vi "TAT-Main.vi"() -> ()   [LabVIEW 2017]
panel:
  in  "Modify SN":bool
  in  "PRINT":bool
  in  "Torque IO Status":bool
  in  "Ass IO Status":bool
  in  "Recipe":bool
  out "error out":errorcluster
  in  "Logout":bool
  in  "Stop":bool
  in  "Create Login":bool
  in  "Reports":bool
  in  "Start":bool
  out "Time":string
  out "Date":string
  in  "Login":bool
  # "RBC ORVM- TRACEABILITY, SCANNING & BARCODE PRINTING"
  # "KAPSE SONS ROBOTICS\n& AUTOMATION"
  # "Contact:-- +91 9325640282"
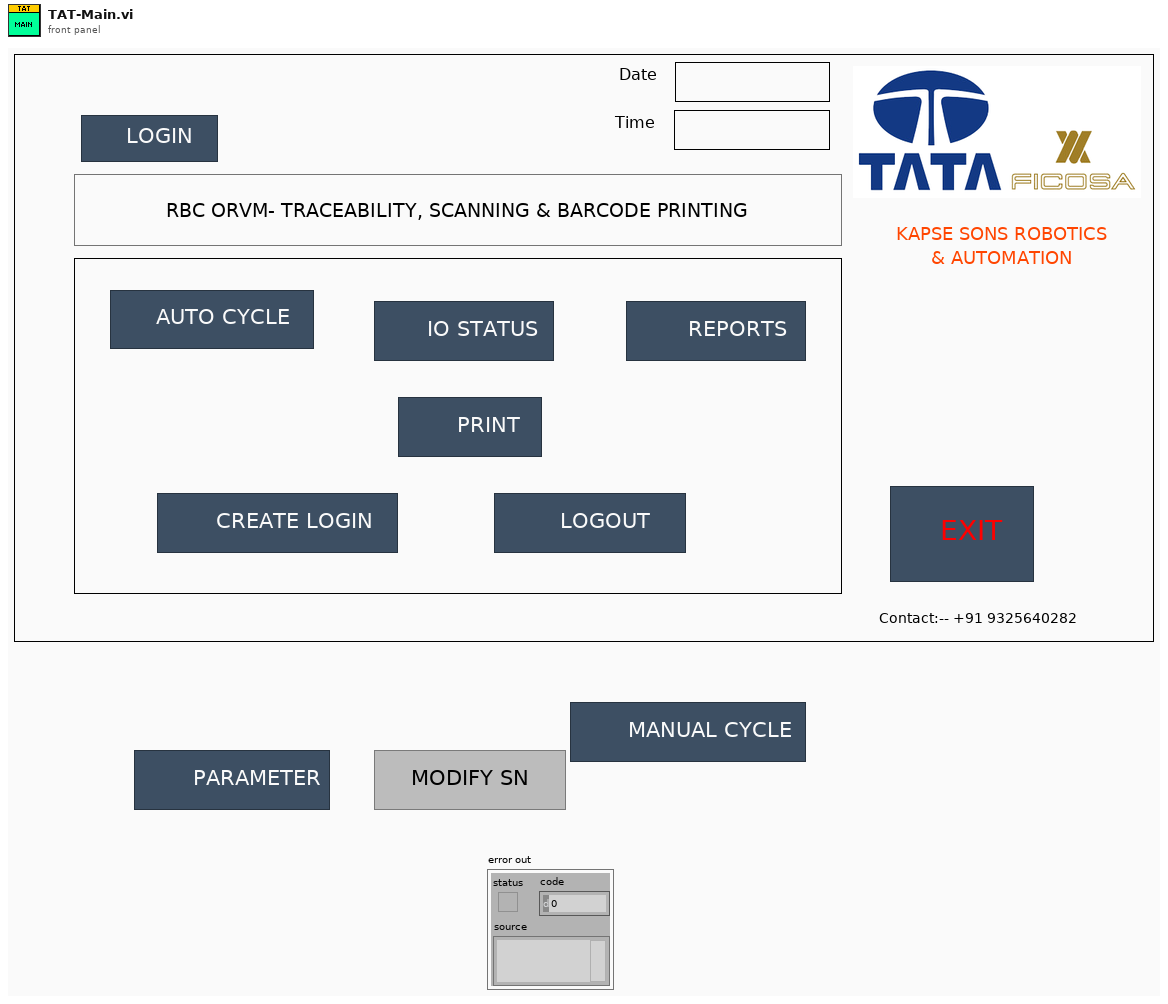
[diagram p1: front panel]
types:
  T1 = enum8{"Enabled", "Disabled", "Disabled and Grayed Out"}
  T2 = enum32{"Invalid", "Standard", "Closed", "Hidden", "Minimized", "Maximized"}
  T3 = enum32{"invalid app kind", "Development System", "Run Time System", "Student Edition", "Embedded LabVIEW", "Evaluation", "Custom"}
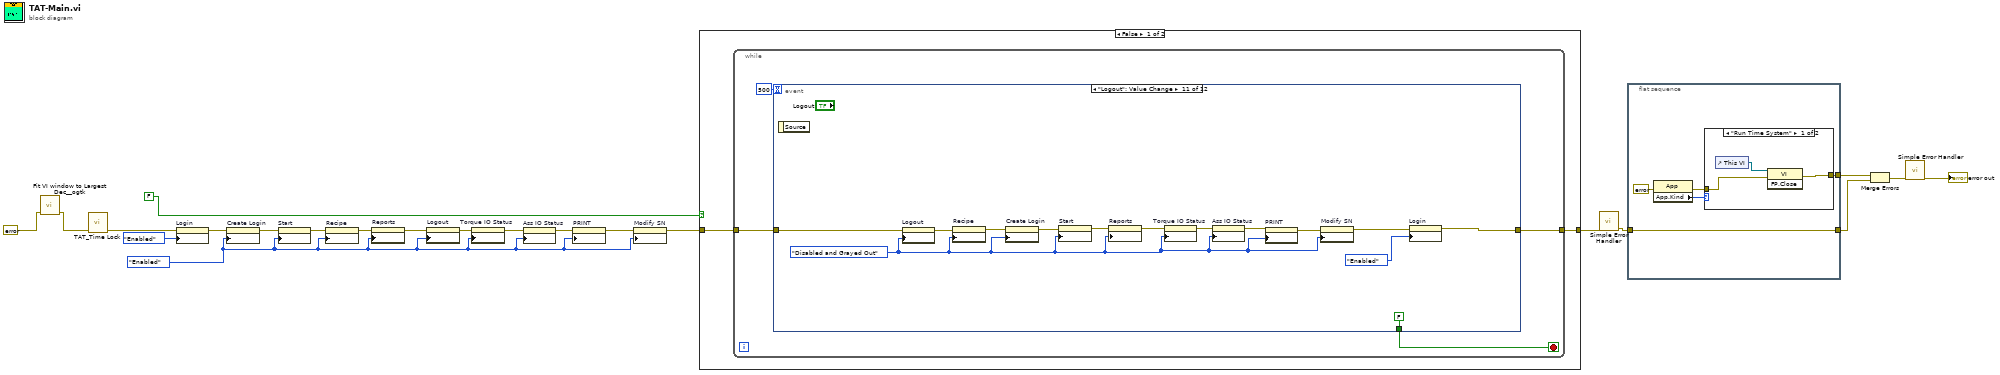
[diagram p0: block diagram]
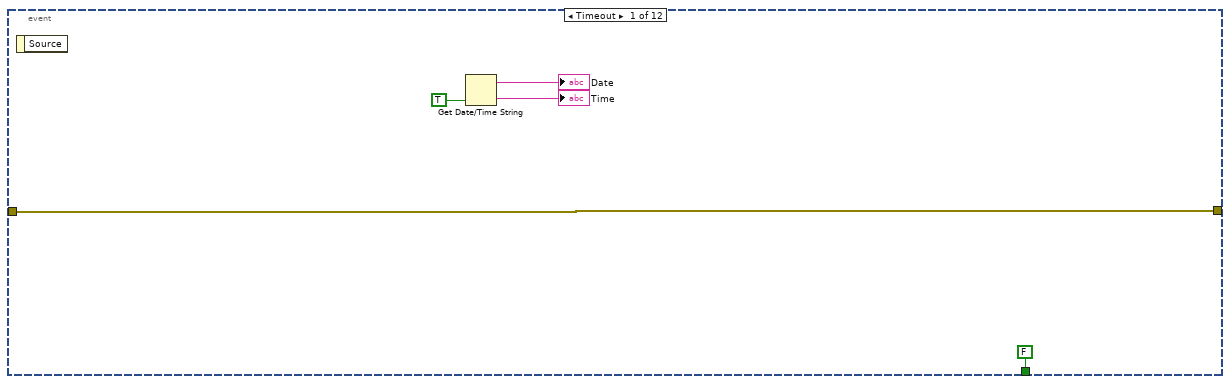
[diagram p3: hidden frame]
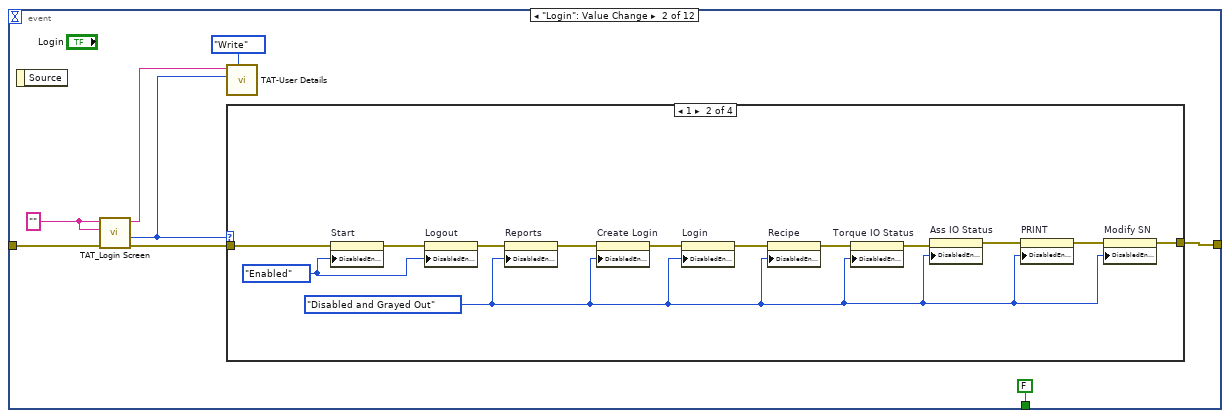
[diagram p4: hidden frame]
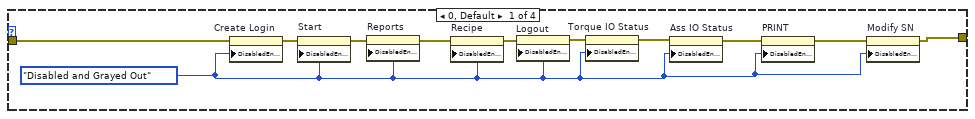
[diagram p5: hidden frame]
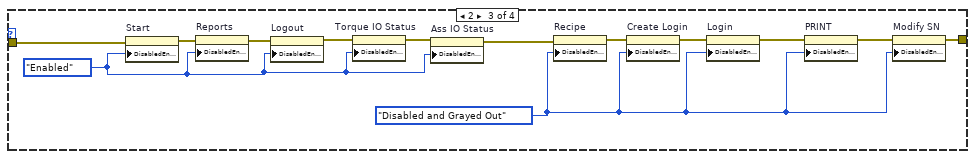
[diagram p6: hidden frame]
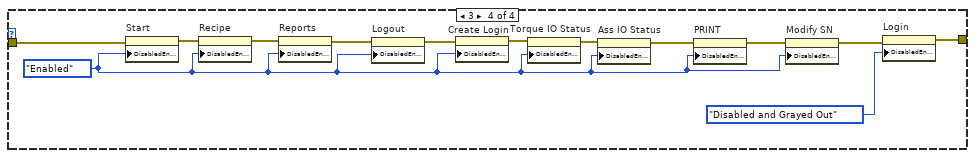
[diagram p7: hidden frame]
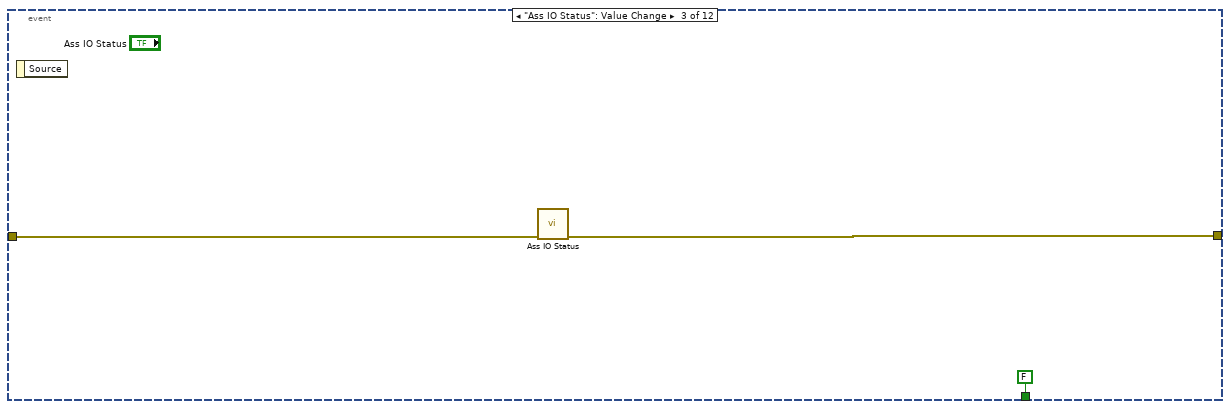
[diagram p8: hidden frame]
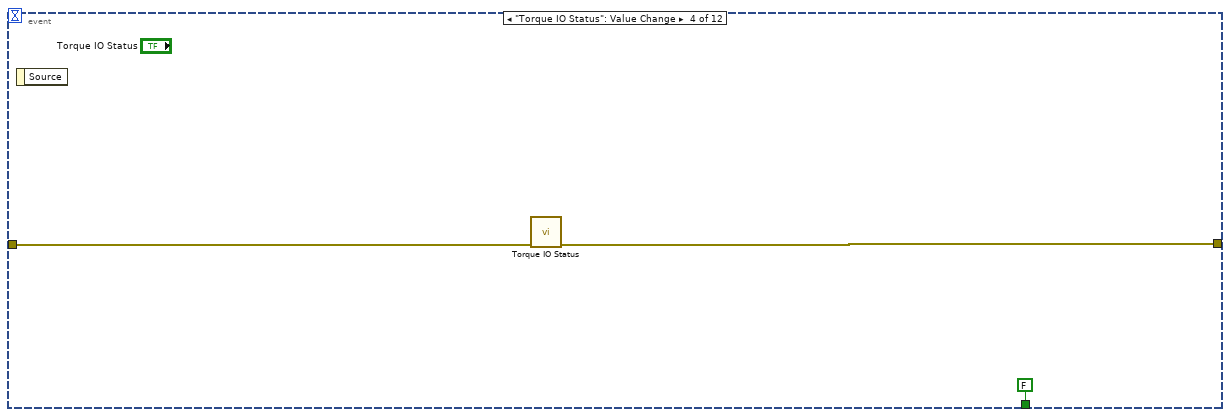
[diagram p9: hidden frame]
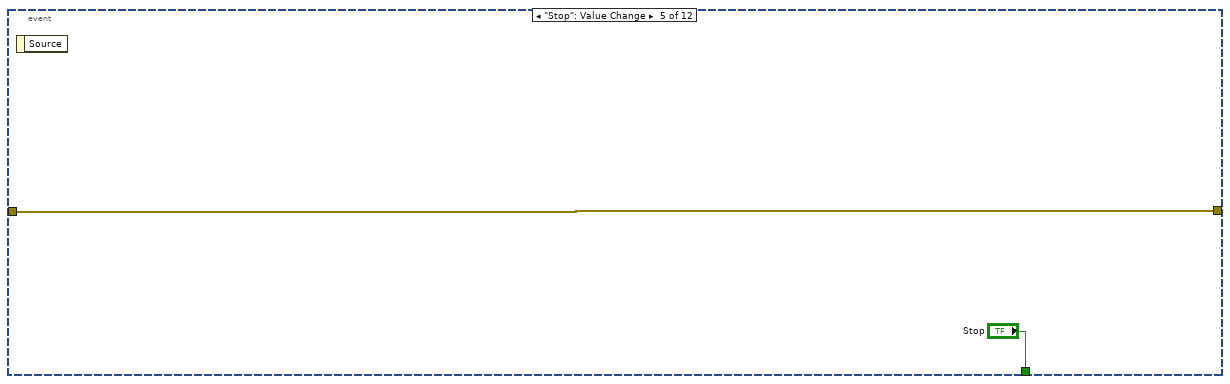
[diagram p10: hidden frame]
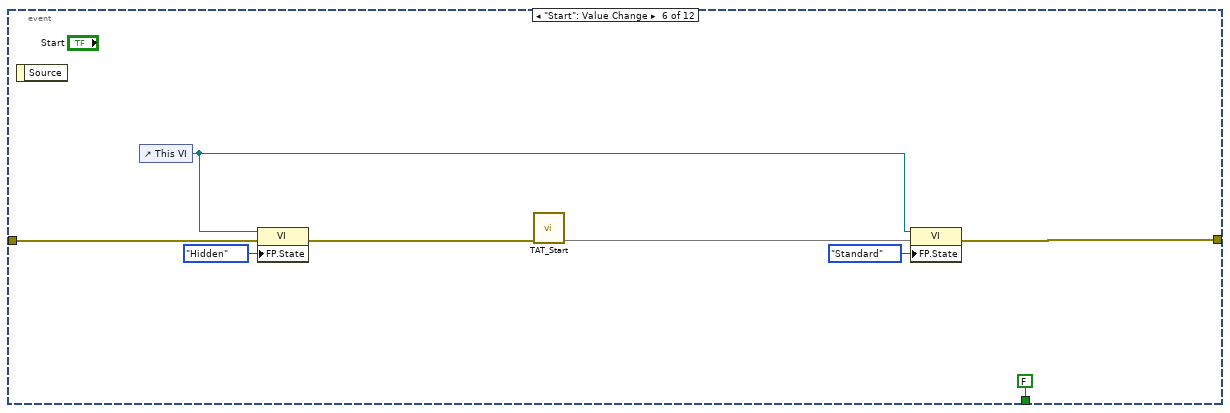
[diagram p11: hidden frame]
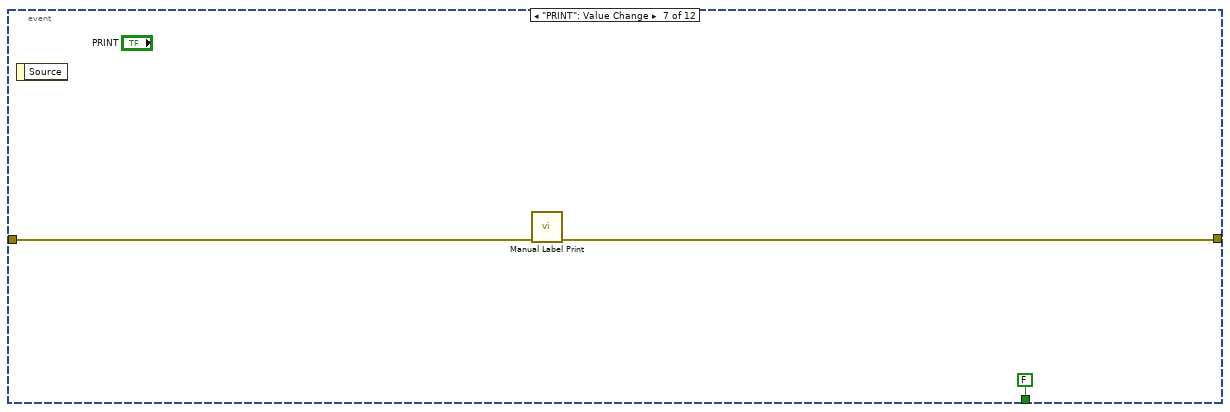
[diagram p12: hidden frame]
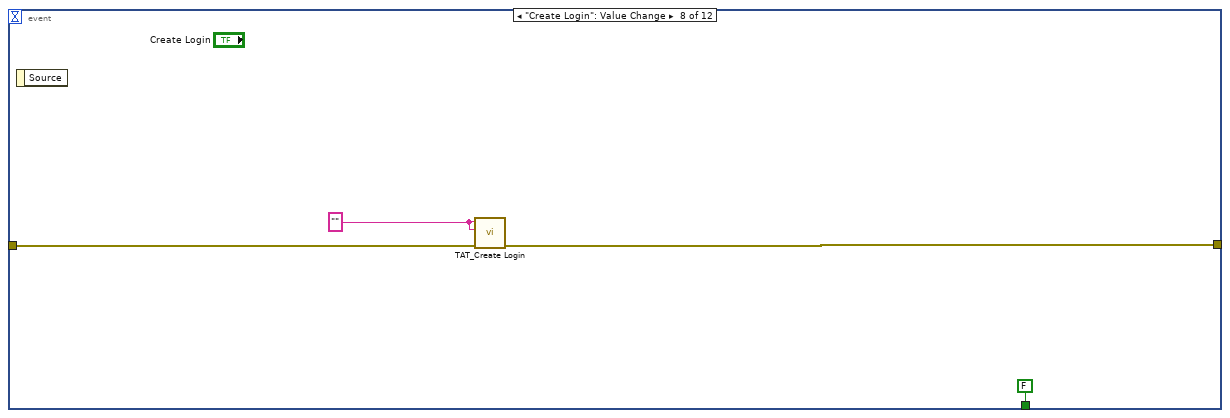
[diagram p13: hidden frame]
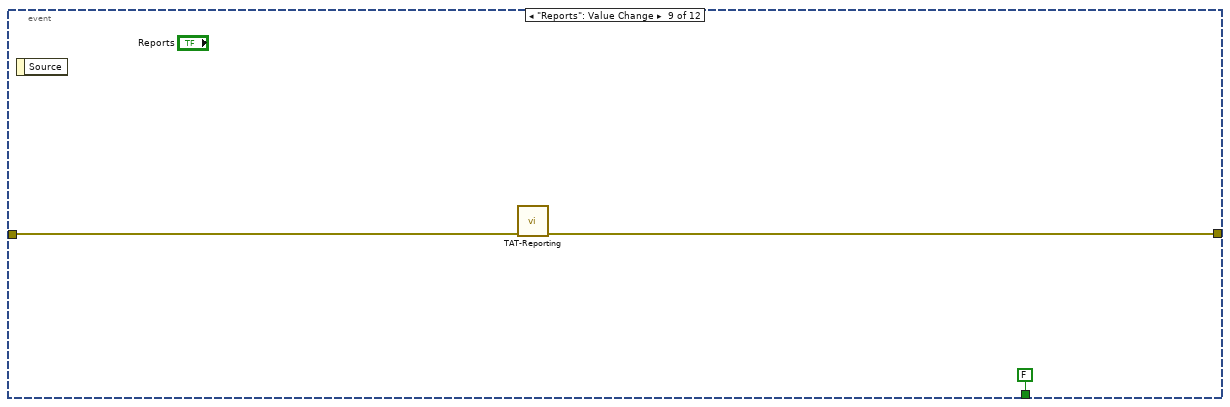
[diagram p14: hidden frame]
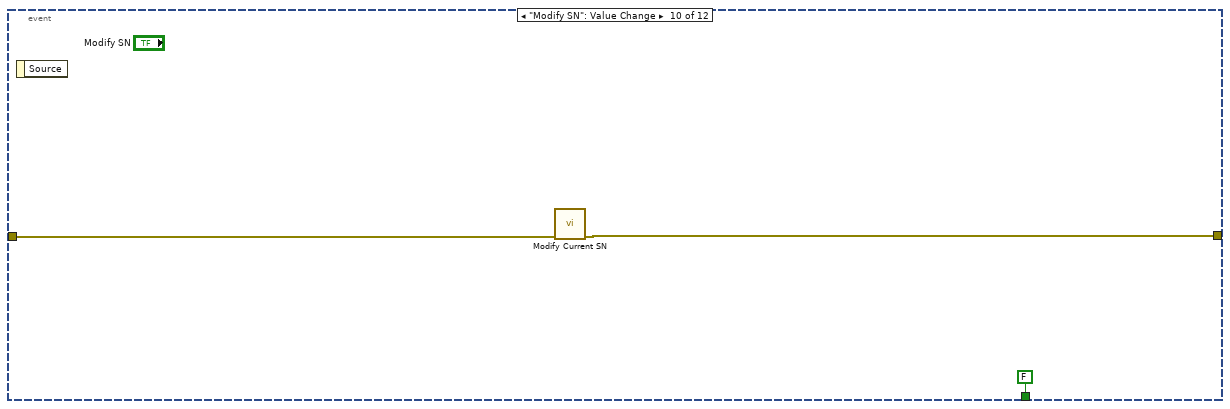
[diagram p15: hidden frame]
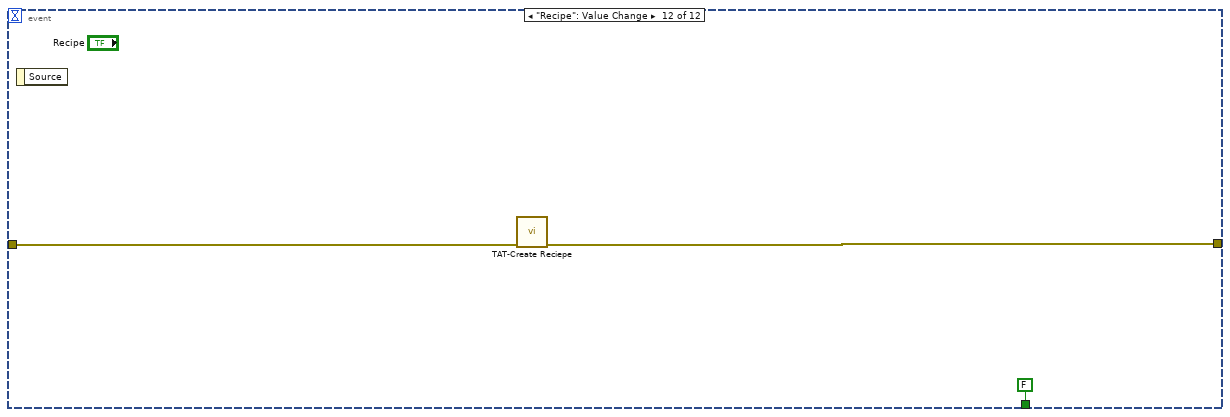
[diagram p16: hidden frame]
diagram:
  w4 = T1."Enabled" ("Disabled")
  n1 = call <userlib>:"Fit VI window to Largest Dec__ogtk.vi"("error in (no error)"=errorcluster {"status"=FALSE, "code"=0, "source"=""} ("error constant")) -> ("error out"=w1:errorcluster)  [unwired: 5 in, 1 out]
  n2 = call "TAT_Time Lock.vi"("error in"=w1) -> ("error out"=w16:errorcluster)  [unwired: 9 in, 1 out]
  n3 = property on="Login" class="Bool"(error in=w16, "DisabledEnum"=T1."Enabled" ("Disabled")) -> (error out=w15:errorcluster)  [unwired: 1 in, 1 out]
  n4 = property on="Create Login" class="Bool"(error in=w15, "DisabledEnum"=w4) -> (error out=w21:errorcluster)  [unwired: 1 in, 1 out]
  n5 = property on="Start" class="Bool"(error in=w21, "DisabledEnum"=w4) -> (error out=w11:errorcluster)  [unwired: 1 in, 1 out]
  n6 = property on="Recipe" class="Bool"(error in=w11, "DisabledEnum"=w4) -> (error out=w10:errorcluster)  [unwired: 1 in, 1 out]
  n7 = property on="Reports" class="Bool"(error in=w10, "DisabledEnum"=w4) -> (error out=w13:errorcluster)  [unwired: 1 in, 1 out]
  n8 = property on="Logout" class="Bool"(error in=w13, "DisabledEnum"=w4) -> (error out=w9:errorcluster)  [unwired: 1 in, 1 out]
  n9 = property on="Torque IO Status" class="Bool"(error in=w9, "DisabledEnum"=w4) -> (error out=w8:errorcluster)  [unwired: 1 in, 1 out]
  n10 = property on="Ass IO Status" class="Bool"(error in=w8, "DisabledEnum"=w4) -> (error out=w7:errorcluster)  [unwired: 1 in, 1 out]
  n11 = property on="PRINT" class="Bool"(error in=w7, "DisabledEnum"=w4) -> (error out=w6:errorcluster)  [unwired: 1 in, 1 out]
  n12 = property on="Modify SN" class="Bool"(error in=w6, "DisabledEnum"=w4) -> (error out=w5:errorcluster)  [unwired: 1 in, 1 out]
  n13 = case shown="False" FALSE {
    tunnel: w5 -> [w24 w138]
    tunnel: [w23 w138] -> w22
    frame False {
      n14 = while {
        tunnel: w24 -> [w27]
        tunnel: [w26] -> w23
        stop <- w25 stop-if-true
        n15 = event shown="[10] \"Logout\": Value Change" {
          selector: _ -> [_ _ _ _ _ _ _ _ _ _ _ _]
          dyn-events: _ -> [_ _ _ _ _ _ _ _ _ _ _ _]
          timeout: 500 -> [_ _ _ _ _ _ _ _ _ _ _ _]
          tunnel: w27 -> [w31 w41 w94 w96 w98 w105 w109 w114 w117 w120 w131 w137]
          tunnel: [w31 w39 w93 w95 w98 w102 w108 w113 w116 w119 w132 w136] -> w26
          tunnel: [FALSE ("Stop") FALSE ("Stop") FALSE ("Stop") FALSE ("Stop") "Stop" FALSE ("Stop") FALSE ("Stop") FALSE ("Stop") FALSE ("Stop") FALSE ("Stop") FALSE ("Stop") FALSE ("Stop")] -> w25
          event Timeout {
            n16 = event-data() -> ()  [unwired: 1 in, 1 out]
            n17 = Get Date/Time String(want seconds? (F)=TRUE) -> (date string=→"Date":string, time string=→"Time":string)  [unwired: 2 in]
          }
          event "Login": Value Change {
            w36 = "" ("User Name")
            n18 = event-data() -> ()  [unwired: 1 in, 1 out]
            n19 = call "TAT_Login Screen.vi"("Error In"=w41, "Password"=w36, "User Name"=w36) -> ("error out"=w40:errorcluster, "Level"=w34:i32, "User Name Out"=w37:string)  [unwired: 5 in, 1 out]
            n20 = call "TAT-User Details.vi"("Enum"=enum16{"Read", "Write"}."Write", "Level In"=w34, "User Name In"=w37) -> ()  [unwired: 7 in, 2 out]
            n21 = case shown="1" w34 {
              tunnel: w40 -> [w50 w65 w78 w91]
              tunnel: [w43 w54 w67 w90] -> w39
              frame 0, Default {
                w42 = T1."Disabled and Grayed Out" ("Disabled")
                n22 = property on="Create Login" class="Bool"(error in=w50, "DisabledEnum"=w42) -> (error out=w52:errorcluster)  [unwired: 1 in, 1 out]
                n23 = property on="Start" class="Bool"(error in=w52, "DisabledEnum"=w42) -> (error out=w51:errorcluster)  [unwired: 1 in, 1 out]
                n24 = property on="Reports" class="Bool"(error in=w51, "DisabledEnum"=w42) -> (error out=w49:errorcluster)  [unwired: 1 in, 1 out]
                n25 = property on="Recipe" class="Bool"(error in=w49, "DisabledEnum"=w42) -> (error out=w48:errorcluster)  [unwired: 1 in, 1 out]
                n26 = property on="Logout" class="Bool"(error in=w48, "DisabledEnum"=w42) -> (error out=w47:errorcluster)  [unwired: 1 in, 1 out]
                n27 = property on="Torque IO Status" class="Bool"(error in=w47, "DisabledEnum"=w42) -> (error out=w46:errorcluster)  [unwired: 1 in, 1 out]
                n28 = property on="Ass IO Status" class="Bool"(error in=w46, "DisabledEnum"=w42) -> (error out=w45:errorcluster)  [unwired: 1 in, 1 out]
                n29 = property on="PRINT" class="Bool"(error in=w45, "DisabledEnum"=w42) -> (error out=w44:errorcluster)  [unwired: 1 in, 1 out]
                n30 = property on="Modify SN" class="Bool"(error in=w44, "DisabledEnum"=w42) -> (error out=w43:errorcluster)  [unwired: 1 in, 1 out]
              }
              frame 1 {
                w53 = T1."Disabled and Grayed Out" ("Disabled")
                w61 = T1."Enabled" ("Disabled")
                n31 = property on="Start" class="Bool"(error in=w65, "DisabledEnum"=w61) -> (error out=w60:errorcluster)  [unwired: 1 in, 1 out]
                n32 = property on="Logout" class="Bool"(error in=w60, "DisabledEnum"=w61) -> (error out=w63:errorcluster)  [unwired: 1 in, 1 out]
                n33 = property on="Reports" class="Bool"(error in=w63, "DisabledEnum"=w53) -> (error out=w64:errorcluster)  [unwired: 1 in, 1 out]
                n34 = property on="Create Login" class="Bool"(error in=w64, "DisabledEnum"=w53) -> (error out=w62:errorcluster)  [unwired: 1 in, 1 out]
                n35 = property on="Login" class="Bool"(error in=w62, "DisabledEnum"=w53) -> (error out=w59:errorcluster)  [unwired: 1 in, 1 out]
                n36 = property on="Recipe" class="Bool"(error in=w59, "DisabledEnum"=w53) -> (error out=w57:errorcluster)  [unwired: 1 in, 1 out]
                n37 = property on="Torque IO Status" class="Bool"(error in=w57, "DisabledEnum"=w53) -> (error out=w58:errorcluster)  [unwired: 1 in, 1 out]
                n38 = property on="Ass IO Status" class="Bool"(error in=w58, "DisabledEnum"=w53) -> (error out=w56:errorcluster)  [unwired: 1 in, 1 out]
                n39 = property on="PRINT" class="Bool"(error in=w56, "DisabledEnum"=w53) -> (error out=w55:errorcluster)  [unwired: 1 in, 1 out]
                n40 = property on="Modify SN" class="Bool"(error in=w55, "DisabledEnum"=w53) -> (error out=w54:errorcluster)  [unwired: 1 in, 1 out]
              }
              frame 2 {
                w66 = T1."Disabled and Grayed Out" ("Disabled")
                w70 = T1."Enabled" ("Disabled")
                n41 = property on="Start" class="Bool"(error in=w78, "DisabledEnum"=w70) -> (error out=w75:errorcluster)  [unwired: 1 in, 1 out]
                n42 = property on="Reports" class="Bool"(error in=w75, "DisabledEnum"=w70) -> (error out=w77:errorcluster)  [unwired: 1 in, 1 out]
                n43 = property on="Logout" class="Bool"(error in=w77, "DisabledEnum"=w70) -> (error out=w72:errorcluster)  [unwired: 1 in, 1 out]
                n44 = property on="Torque IO Status" class="Bool"(error in=w72, "DisabledEnum"=w70) -> (error out=w73:errorcluster)  [unwired: 1 in, 1 out]
                n45 = property on="Ass IO Status" class="Bool"(error in=w73, "DisabledEnum"=w70) -> (error out=w71:errorcluster)  [unwired: 1 in, 1 out]
                n46 = property on="Recipe" class="Bool"(error in=w71, "DisabledEnum"=w66) -> (error out=w74:errorcluster)  [unwired: 1 in, 1 out]
                n47 = property on="Create Login" class="Bool"(error in=w74, "DisabledEnum"=w66) -> (error out=w76:errorcluster)  [unwired: 1 in, 1 out]
                n48 = property on="Login" class="Bool"(error in=w76, "DisabledEnum"=w66) -> (error out=w69:errorcluster)  [unwired: 1 in, 1 out]
                n49 = property on="PRINT" class="Bool"(error in=w69, "DisabledEnum"=w66) -> (error out=w68:errorcluster)  [unwired: 1 in, 1 out]
                n50 = property on="Modify SN" class="Bool"(error in=w68, "DisabledEnum"=w66) -> (error out=w67:errorcluster)  [unwired: 1 in, 1 out]
              }
              frame 3 {
                w79 = T1."Enabled" ("Disabled")
                n51 = property on="Start" class="Bool"(error in=w91, "DisabledEnum"=w79) -> (error out=w86:errorcluster)  [unwired: 1 in, 1 out]
                n52 = property on="Recipe" class="Bool"(error in=w86, "DisabledEnum"=w79) -> (error out=w85:errorcluster)  [unwired: 1 in, 1 out]
                n53 = property on="Reports" class="Bool"(error in=w85, "DisabledEnum"=w79) -> (error out=w88:errorcluster)  [unwired: 1 in, 1 out]
                n54 = property on="Logout" class="Bool"(error in=w88, "DisabledEnum"=w79) -> (error out=w87:errorcluster)  [unwired: 1 in, 1 out]
                n55 = property on="Create Login" class="Bool"(error in=w87, "DisabledEnum"=w79) -> (error out=w84:errorcluster)  [unwired: 1 in, 1 out]
                n56 = property on="Torque IO Status" class="Bool"(error in=w84, "DisabledEnum"=w79) -> (error out=w83:errorcluster)  [unwired: 1 in, 1 out]
                n57 = property on="Ass IO Status" class="Bool"(error in=w83, "DisabledEnum"=w79) -> (error out=w82:errorcluster)  [unwired: 1 in, 1 out]
                n58 = property on="PRINT" class="Bool"(error in=w82, "DisabledEnum"=w79) -> (error out=w81:errorcluster)  [unwired: 1 in, 1 out]
                n59 = property on="Modify SN" class="Bool"(error in=w81, "DisabledEnum"=w79) -> (error out=w80:errorcluster)  [unwired: 1 in, 1 out]
                n60 = property on="Login" class="Bool"(error in=w80, "DisabledEnum"=T1."Disabled and Grayed Out" ("Disabled")) -> (error out=w90:errorcluster)  [unwired: 1 in, 1 out]
              }
            }
          }
          event "Ass IO Status": Value Change {
            n61 = event-data() -> ()  [unwired: 1 in, 1 out]
            n62 = call "Ass IO Status.vi"("error in (no error)"=w94) -> ("error out"=w93:errorcluster)  [unwired: 10 in]
          }
          event "Torque IO Status": Value Change {
            n63 = event-data() -> ()  [unwired: 1 in, 1 out]
            n64 = call "Torque IO Status.vi"("error in (no error)"=w96) -> ("error out"=w95:errorcluster)  [unwired: 10 in]
          }
          event "Stop": Value Change {
            n65 = event-data() -> ()  [unwired: 1 in, 1 out]
          }
          event "Start": Value Change {
            n66 = event-data() -> ()  [unwired: 1 in, 1 out]
            n67 = control-ref of="This VI"() -> (w103:refnum<vi>)
            n68 = property class="VI"(reference=w103, error in=w105, "FP.State"=T2."Hidden" ("Front Panel Window:State")) -> (error out=w101:errorcluster)  [unwired: 1 out]
            n69 = call "TAT_Start.vi"("error In"=w101) -> (0:w100)  [unwired: 10 in]
            n70 = property class="VI"(reference=w103, error in=w100, "FP.State"=T2."Standard" ("Front Panel Window:State")) -> (error out=w102:errorcluster)  [unwired: 1 out]
          }
          event "PRINT": Value Change {
            n71 = event-data() -> ()  [unwired: 1 in, 1 out]
            n72 = call "Manual Label Print.vi"("error in (no error)"=w109) -> ("error out"=w108:errorcluster)  [unwired: 10 in]
          }
          event "Create Login": Value Change {
            w112 = "" ("User Name")
            n73 = event-data() -> ()  [unwired: 1 in, 1 out]
            n74 = call "TAT_Create Login.vi"("Error In"=w114, "Password"=w112, "User Name"=w112) -> ("error out"=w113:errorcluster)  [unwired: 6 in]
          }
          event "Reports": Value Change {
            n75 = event-data() -> ()  [unwired: 1 in, 1 out]
            n76 = call "TAT-Reporting.vi"("error in (no error)"=w117) -> ("error out"=w116:errorcluster)  [unwired: 10 in]
          }
          event "Modify SN": Value Change {
            n77 = event-data() -> ()  [unwired: 1 in, 1 out]
            n78 = call "Modify Current SN.vi"("error in (no error)"=w120) -> ("error out"=w119:errorcluster)  [unwired: 10 in]
          }
          event "Logout": Value Change {
            w121 = T1."Disabled and Grayed Out" ("Disabled")
            n79 = event-data() -> ()  [unwired: 1 in, 1 out]
            n80 = property on="Logout" class="Bool"(error in=w131, "DisabledEnum"=w121) -> (error out=w129:errorcluster)  [unwired: 1 in, 1 out]
            n81 = property on="Recipe" class="Bool"(error in=w129, "DisabledEnum"=w121) -> (error out=w128:errorcluster)  [unwired: 1 in, 1 out]
            n82 = property on="Create Login" class="Bool"(error in=w128, "DisabledEnum"=w121) -> (error out=w134:errorcluster)  [unwired: 1 in, 1 out]
            n83 = property on="Start" class="Bool"(error in=w134, "DisabledEnum"=w121) -> (error out=w133:errorcluster)  [unwired: 1 in, 1 out]
            n84 = property on="Reports" class="Bool"(error in=w133, "DisabledEnum"=w121) -> (error out=w126:errorcluster)  [unwired: 1 in, 1 out]
            n85 = property on="Torque IO Status" class="Bool"(error in=w126, "DisabledEnum"=w121) -> (error out=w127:errorcluster)  [unwired: 1 in, 1 out]
            n86 = property on="Ass IO Status" class="Bool"(error in=w127, "DisabledEnum"=w121) -> (error out=w124:errorcluster)  [unwired: 1 in, 1 out]
            n87 = property on="PRINT" class="Bool"(error in=w124, "DisabledEnum"=w121) -> (error out=w123:errorcluster)  [unwired: 1 in, 1 out]
            n88 = property on="Modify SN" class="Bool"(error in=w123, "DisabledEnum"=w121) -> (error out=w122:errorcluster)  [unwired: 1 in, 1 out]
            n89 = property on="Login" class="Bool"(error in=w122, "DisabledEnum"=T1."Enabled" ("Disabled")) -> (error out=w132:errorcluster)  [unwired: 1 in, 1 out]
          }
          event "Recipe": Value Change {
            n90 = event-data() -> ()  [unwired: 1 in, 1 out]
            n91 = call "TAT-Create Reciepe.vi"("Error In"=w137) -> ("error out"=w136:errorcluster)  [unwired: 10 in]
          }
        }
      }
    }
    frame True {
    }
  }
  n92 = call <vilib>:"Simple Error Handler.vi"("error in (no error)"=w22) -> ("error out"=w17:errorcluster)  [unwired: 4 in, 4 out]
  n93 = flat-sequence {
    tunnel: [w140] -> w20
    tunnel: [w139] -> w18
    tunnel: w17 -> [w139]
    frame #0 {
      n94 = property class="App"(error in=errorcluster {"status"=FALSE, "code"=0, "source"=""} ("error in (no error)")) -> (error out=w142:errorcluster, "App.Kind"=w143:T3)  [unwired: 1 in, 1 out]
      n95 = case shown="\"Run Time System\"" w143 {
        tunnel: w142 -> [w145 w147]
        tunnel: [w144 w147] -> w140
        frame "Run Time System" {
          n96 = control-ref of="This VI"() -> (w146:refnum<vi>)
          n97 = invoke class="VI" method="FP.Close"(reference=w146, error in=w145) -> (error out=w144:errorcluster)  [unwired: 1 in, 2 out]
        }
        frame "Development System", Default {
        }
      }
    }
  }
  n98 = Merge Errors(w20, w18) -> (w19:errorcluster)
  n99 = call <vilib>:"Simple Error Handler.vi"("error in (no error)"=w19) -> ("error out"=→"error out":errorcluster)  [unwired: 4 in, 4 out]
